vi "ExecuteOperation.vi"(8 "error in":errorcluster, 9 "Operation Path":path, 10 "Logger information":T1={"Log File Path"="", "Verbosity"=enum."Default", "Append to log file?"=FALSE}, 11 "Inputs":string[](array[string])) -> (0 "error out":errorcluster, 2 "Output/Failure messages":string, 3 "CLI Process Return Code":i32)   [LabVIEW 2014]
uses:
  Utilities/Logger/LoggerCore.ctl
  Utilities/Verbosity.ctl
  Utilities/Logger/Logger.lvclass
  CoreOperation/CoreOperation.lvclass
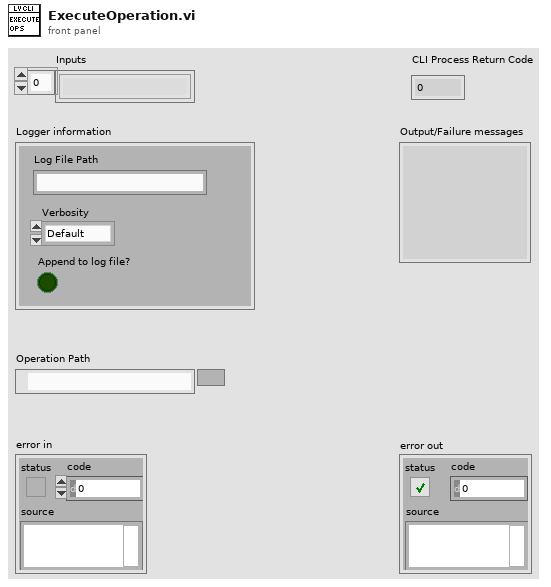
[diagram p1: front panel]
types:
  T1 = typedef "Logger.lvclass/LoggerCore.ctl" = cluster{"Log File Path":string, "Verbosity":T2, "Append to log file?":bool}
  T2 = typedef "Verbosity.ctl" = enum16{"Minimal", "Default", "Detailed", "Diagnostic"}
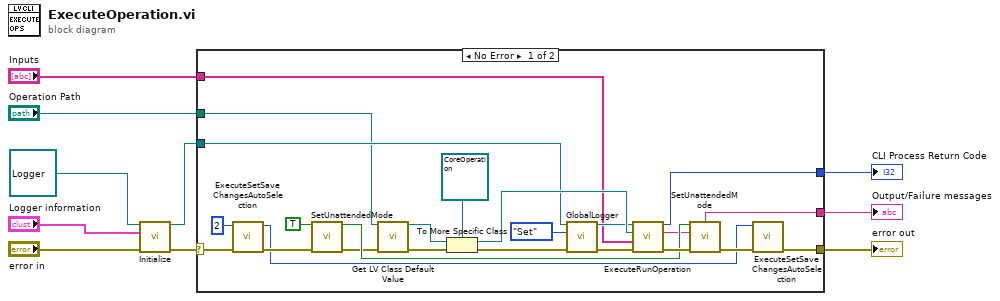
[diagram p0: block diagram]
diagram:
  n1 = call "Initialize.vi"("error in (no error)"="error in", "Logger information"="Logger information", "Logger in"=refnum<class "Logger.lvclass"> refnum ("Logger.lvclass")) -> ("error out"=w2:errorcluster, "Logger out"=w1:refnum<class "Logger.lvclass">)  [unwired: 7 in]
  n2 = case shown="No Error" w2 {
    selector: w2 -> [w29 w34]
    tunnel: "Inputs" -> [w17 _]
    tunnel: [w13 w34] -> w9
    tunnel: w1 -> [w19 _]
    tunnel: "Operation Path" -> [w15 _]
    tunnel: [w24 _] -> w7
    tunnel: [w23 _] -> w6
    frame No Error {
      n3 = call "ExecuteSetSaveChangesAutoSelection.vi"("error in (no error)"=w29, "New SaveChangesAutoSelection value"=2) -> ("error out"=w14:errorcluster, "Previous SaveChangesAutoSelection value"=w12:i32)  [unwired: 8 in]
      n4 = call "SetUnattendedMode.vi"("error in (no error)"=w14, "New value"=TRUE ("Set to")) -> ("error out"=w16:errorcluster, "Previous value"=w26:bool)  [unwired: 8 in]
      n5 = call <vilib>:"Get LV Class Default Value.vi"("error in (no error)"=w16, "class path"=w15) -> ("error out"=w31:errorcluster, "object"=w32:refnum<class>)  [unwired: 8 in]
      n6 = To More Specific Class(target class=refnum<class "CoreOperation.lvclass"> refnum ("CoreOperation.lvclass"), reference=w32, error in=w31) -> (specific class reference=w30:refnum<class "CoreOperation.lvclass">, error out=w20:errorcluster)
      n7 = call "GlobalLogger.vi"("error in (no error)"=w20, "Enum"=enum16{"Get", "Set"}."Set", "Logger in"=w19) -> ("error out"=w21:errorcluster, "Logger"=w22:refnum<class "Logger.lvclass">)  [unwired: 7 in]
      n8 = call "ExecuteRunOperation.vi"("error in (no error)"=w21, "Inputs"=w17, "CoreOperation.lvclass"=w30, "Logger in"=w22) -> ("error out"=w27:errorcluster, "Output/Failure"=w23:string, "CLI Process Return Code"=w24:i32)  [unwired: 5 in]
      n9 = call "SetUnattendedMode.vi"("error in (no error)"=w27, "New value"=w26) -> ("error out"=w25:errorcluster)  [unwired: 8 in, 1 out]
      n10 = call "ExecuteSetSaveChangesAutoSelection.vi"("error in (no error)"=w25, "New SaveChangesAutoSelection value"=w12) -> ("error out"=w13:errorcluster)  [unwired: 8 in, 1 out]
    }
    frame Error {
    }
  }
  "error out" <- w9
  "CLI Process Return Code" <- w7
  "Output/Failure messages" <- w6
